vi "replacefilename.vi"(7 "new filenamePART":string="dfgdfgdfgd", 11 "filename":string="Scan035_StagingMagSpec_014_Ebeam.png") -> (3 "filename out":string)   [LabVIEW 2013]
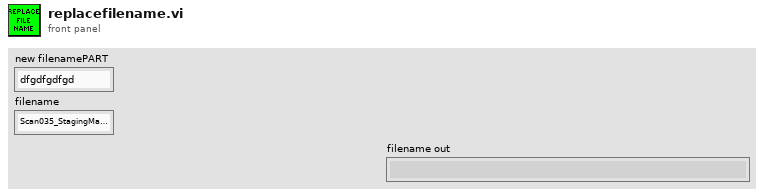
[diagram p1: front panel]
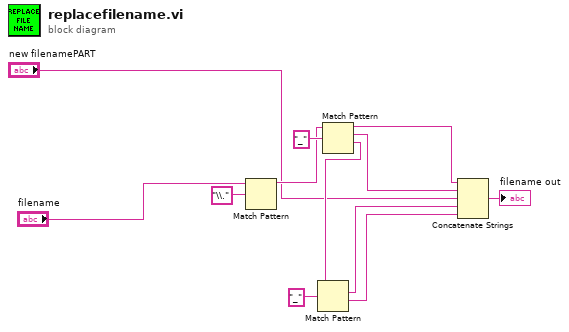
[diagram p0: block diagram]
diagram:
  n1 = Match Pattern(string="filename", regular expression="\\.") -> (before substring=w5:string)  [unwired: 1 in, 3 out]
  n2 = Match Pattern(string=w5, regular expression="_") -> (before substring=w3:string, match substring=w2:string, after substring=w4:string)  [unwired: 1 in, 1 out]
  n3 = Match Pattern(string=w4, regular expression="_") -> (match substring=w9:string, after substring=w8:string)  [unwired: 1 in, 2 out]
  n4 = Concatenate Strings(w3, w2, "new filenamePART", w9, w8) -> (→"filename out":string)
